vi "Visible Scrollbar.vi"(8 "error in (no error)":errorcluster, 10 "scrollbars":enum8{"hide", "show"}(ring), 11 "GObject in":refnum<vi>) -> (0 "error out":errorcluster, 1 "was scrollbars visible?":enum8{"hide", "show"}(ring), 2 "has scrollbars?":bool, 3 "GObject out":refnum<vi>)   [LabVIEW 2019, in "Builtins.lvlib"]
doc: "Shows or hides the scrollbars if it exists.\n\nCreated by: Ryan Pacini"
uses:
  Builtins.lvlib
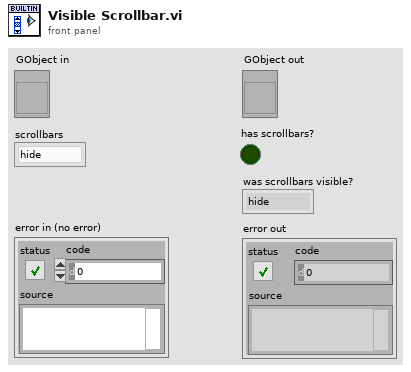
[diagram p1: front panel]
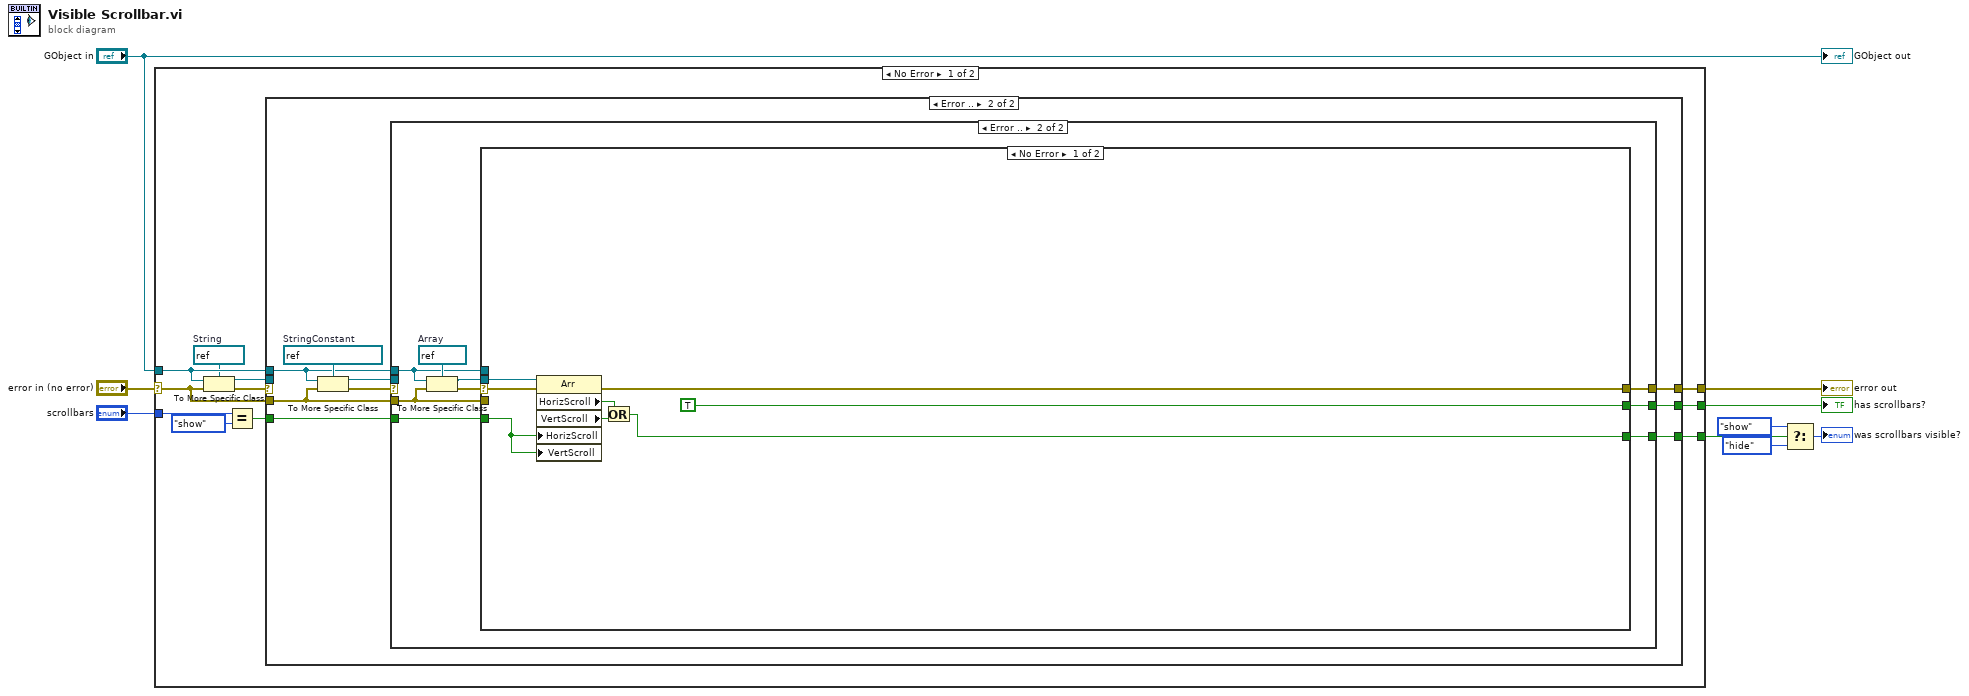
[diagram p0: block diagram]
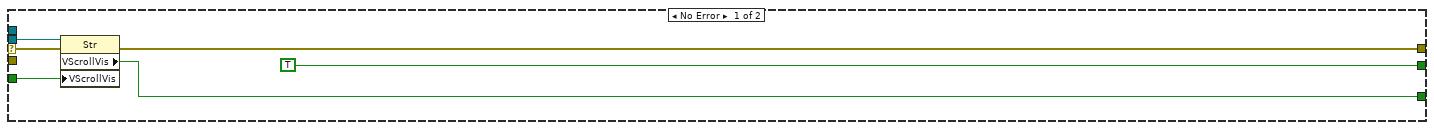
[diagram p2: hidden frame]
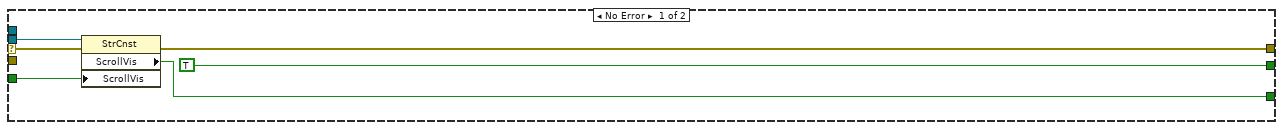
[diagram p3: hidden frame]
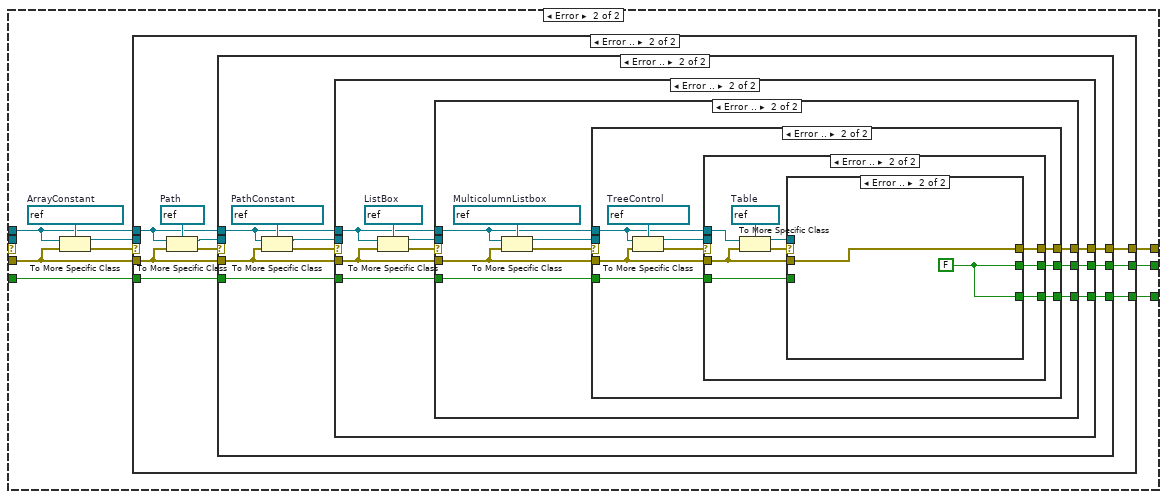
[diagram p4: hidden frame]
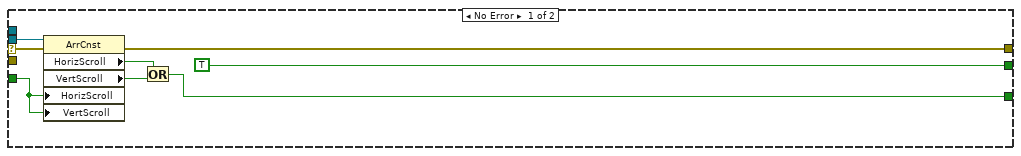
[diagram p5: hidden frame]
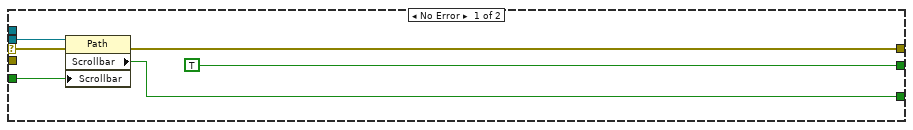
[diagram p6: hidden frame]
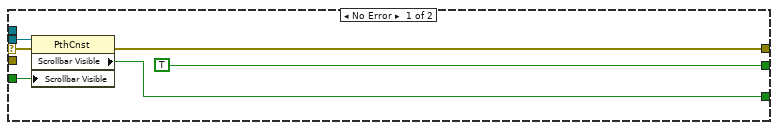
[diagram p7: hidden frame]
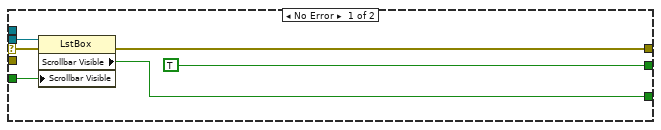
[diagram p8: hidden frame]
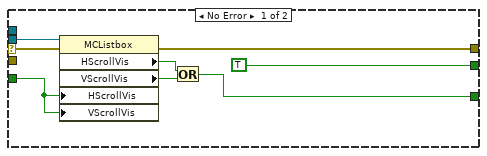
[diagram p9: hidden frame]
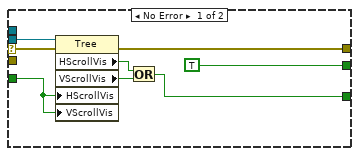
[diagram p10: hidden frame]
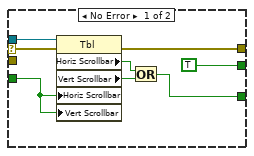
[diagram p11: hidden frame]
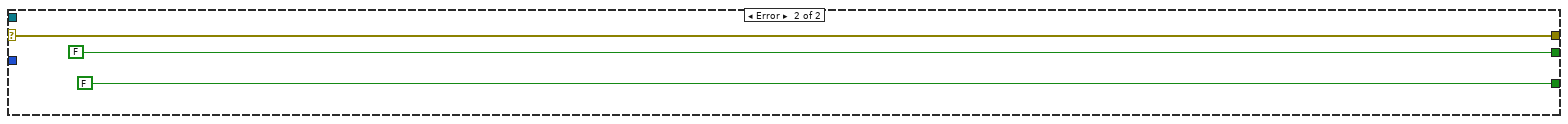
[diagram p12: hidden frame]
diagram:
  n1 = case shown="No Error" "error in (no error)" {
    selector: "error in (no error)" -> [w18 w176]
    tunnel: "GObject in" -> [w19 _]
    tunnel: "scrollbars" -> [w15 _]
    tunnel: [w20 w176] -> w7
    tunnel: [w17 FALSE] -> w6
    tunnel: [w16 FALSE ("ScrollVis")] -> w4
    frame No Error {
      w12 = refnum<vi> refnum  # String
      n2 = To More Specific Class(target class=w12, reference=w19, error in=w18) -> (specific class reference=w10:refnum<vi>, error out=w11:errorcluster)
      n3 = Equal?(x=w15, y=enum8{"hide", "show"}."show") -> (x = y?=w13:bool)
      n4 = case shown="Error .." w11 {
        selector: w11 -> [w25 _]
        tunnel: w10 -> [w24 _]
        tunnel: w13 -> [w23 w32]
        tunnel: [w22 w30] -> w20
        tunnel: w18 -> [_ w29]
        tunnel: [TRUE w31] -> w17
        tunnel: w19 -> [_ w27]
        tunnel: [w21 w28] -> w16
        frame No Error {
          n5 = property class="Str"(reference=w24, error in=w25, "VScrollVis"=w23) -> (error out=w22:errorcluster, "VScrollVis"=w21:bool)  [unwired: 1 out]
        }
        frame Error {
          w35 = refnum<vi> refnum  # StringConstant
          n6 = To More Specific Class(target class=w35, reference=w27, error in=w29) -> (specific class reference=w33:refnum<vi>, error out=w34:errorcluster)
          n7 = case shown="Error .." w34 {
            selector: w34 -> [w41 _]
            tunnel: w33 -> [w40 _]
            tunnel: w32 -> [w39 w45]
            tunnel: [TRUE w50] -> w31
            tunnel: [w37 w44] -> w30
            tunnel: w29 -> [_ w43]
            tunnel: [w36 w49] -> w28
            tunnel: w27 -> [_ w42]
            frame No Error {
              n8 = property class="StrCnst"(reference=w40, error in=w41, "ScrollVis"=w39) -> (error out=w37:errorcluster, "ScrollVis"=w36:bool)  [unwired: 1 out]
            }
            frame Error {
              w48 = refnum<vi> refnum  # Array
              n9 = To More Specific Class(target class=w48, reference=w42, error in=w43) -> (specific class reference=w46:refnum<vi>, error out=w47:errorcluster)
              n10 = case shown="No Error" w47 {
                selector: w47 -> [w57 _]
                tunnel: [TRUE w62] -> w50
                tunnel: [w53 w63] -> w49
                tunnel: w46 -> [w56 _]
                tunnel: w45 -> [w52 w64]
                tunnel: [w51 w60] -> w44
                tunnel: w43 -> [_ w61]
                tunnel: w42 -> [_ w59]
                frame No Error {
                  n11 = property class="Arr"(reference=w56, error in=w57, "HorizScroll"=w52, "VertScroll"=w52) -> (error out=w51:errorcluster, "HorizScroll"=w55:bool, "VertScroll"=w54:bool)  [unwired: 1 out]
                  n12 = Or(x=w55, y=w54) -> (x .or. y?=w53:bool)
                }
                frame Error {
                  w67 = refnum<vi> refnum  # ArrayConstant
                  n13 = To More Specific Class(target class=w67, reference=w59, error in=w61) -> (specific class reference=w65:refnum<vi>, error out=w66:errorcluster)
                  n14 = case shown="Error .." w66 {
                    selector: w66 -> [w73 _]
                    tunnel: w65 -> [w72 _]
                    tunnel: w64 -> [w71 w79]
                    tunnel: [w70 w81] -> w63
                    tunnel: [TRUE w80] -> w62
                    tunnel: w61 -> [_ w77]
                    tunnel: [w68 w78] -> w60
                    tunnel: w59 -> [_ w76]
                    frame No Error {
                      n15 = property class="ArrCnst"(reference=w72, error in=w73, "HorizScroll"=w71, "VertScroll"=w71) -> (error out=w68:errorcluster, "HorizScroll"=w75:bool, "VertScroll"=w74:bool)  [unwired: 1 out]
                      n16 = Or(x=w75, y=w74) -> (x .or. y?=w70:bool)
                    }
                    frame Error {
                      w84 = refnum<vi> refnum  # Path
                      n17 = To More Specific Class(target class=w84, reference=w76, error in=w77) -> (specific class reference=w82:refnum<vi>, error out=w83:errorcluster)
                      n18 = case shown="Error .." w83 {
                        selector: w83 -> [w90 _]
                        tunnel: w82 -> [w89 _]
                        tunnel: [w88 w96] -> w81
                        tunnel: [TRUE w94] -> w80
                        tunnel: w79 -> [w86 w95]
                        tunnel: [w85 w93] -> w78
                        tunnel: w77 -> [_ w92]
                        tunnel: w76 -> [_ w91]
                        frame No Error {
                          n19 = property class="Path"(reference=w89, error in=w90, "Scrollbar"=w86) -> (error out=w85:errorcluster, "Scrollbar"=w88:bool)  [unwired: 1 out]
                        }
                        frame Error {
                          w99 = refnum<vi> refnum  # PathConstant
                          n20 = To More Specific Class(target class=w99, reference=w91, error in=w92) -> (specific class reference=w97:refnum<vi>, error out=w98:errorcluster)
                          n21 = case shown="Error .." w98 {
                            selector: w98 -> [w105 _]
                            tunnel: w97 -> [w104 _]
                            tunnel: [w103 w110] -> w96
                            tunnel: w95 -> [w102 w111]
                            tunnel: [TRUE w109] -> w94
                            tunnel: [w100 w108] -> w93
                            tunnel: w92 -> [_ w107]
                            tunnel: w91 -> [_ w106]
                            frame No Error {
                              n22 = property class="PthCnst"(reference=w104, error in=w105, "Scrollbar Visible"=w102) -> (error out=w100:errorcluster, "Scrollbar Visible"=w103:bool)  [unwired: 1 out]
                            }
                            frame Error {
                              w114 = refnum<vi> refnum  # ListBox
                              n23 = To More Specific Class(target class=w114, reference=w106, error in=w107) -> (specific class reference=w112:refnum<vi>, error out=w113:errorcluster)
                              n24 = case shown="Error .." w113 {
                                selector: w113 -> [w120 _]
                                tunnel: w112 -> [w119 _]
                                tunnel: w111 -> [w118 w123]
                                tunnel: [w117 w126] -> w110
                                tunnel: [TRUE w125] -> w109
                                tunnel: [w115 w124] -> w108
                                tunnel: w107 -> [_ w122]
                                tunnel: w106 -> [_ w121]
                                frame No Error {
                                n25 = property class="LstBox"(reference=w119, error in=w120, "Scrollbar Visible"=w118) -> (error out=w115:errorcluster, "Scrollbar Visible"=w117:bool)  [unwired: 1 out]
                                }
                                frame Error {
                                w129 = refnum<vi> refnum  # MulticolumnListbox
                                n26 = To More Specific Class(target class=w129, reference=w121, error in=w122) -> (specific class reference=w127:refnum<vi>, error out=w128:errorcluster)
                                n27 = case shown="Error .." w128 {
                                selector: w128 -> [w137 _]
                                tunnel: w127 -> [w136 _]
                                tunnel: [w133 w143] -> w126
                                tunnel: [TRUE w142] -> w125
                                tunnel: [w131 w141] -> w124
                                tunnel: w123 -> [w130 w140]
                                tunnel: w122 -> [_ w139]
                                tunnel: w121 -> [_ w138]
                                frame No Error {
                                n28 = property class="MCListbox"(reference=w136, error in=w137, "HScrollVis"=w130, "VScrollVis"=w130) -> (error out=w131:errorcluster, "HScrollVis"=w135:bool, "VScrollVis"=w134:bool)  [unwired: 1 out]
                                n29 = Or(x=w135, y=w134) -> (x .or. y?=w133:bool)
                                }
                                frame Error {
                                w146 = refnum<vi> refnum  # TreeControl
                                n30 = To More Specific Class(target class=w146, reference=w138, error in=w139) -> (specific class reference=w144:refnum<vi>, error out=w145:errorcluster)
                                n31 = case shown="Error .." w145 {
                                selector: w145 -> [w154 _]
                                tunnel: w144 -> [w153 _]
                                tunnel: [w150 w158] -> w143
                                tunnel: [TRUE w157] -> w142
                                tunnel: [w148 w156] -> w141
                                tunnel: w140 -> [w147 w159]
                                tunnel: w139 -> [_ w155]
                                tunnel: w138 -> [_ w162]
                                frame No Error {
                                n32 = property class="Tree"(reference=w153, error in=w154, "HScrollVis"=w147, "VScrollVis"=w147) -> (error out=w148:errorcluster, "HScrollVis"=w151:bool, "VScrollVis"=w152:bool)  [unwired: 1 out]
                                n33 = Or(x=w151, y=w152) -> (x .or. y?=w150:bool)
                                }
                                frame Error {
                                w163 = refnum<vi> refnum  # Table
                                n34 = To More Specific Class(target class=w163, reference=w162, error in=w155) -> (specific class reference=w160:refnum<vi>, error out=w161:errorcluster)
                                n35 = case shown="Error .." w161 {
                                selector: w161 -> [w169 _]
                                tunnel: w160 -> [w168 _]
                                tunnel: w159 -> [w167 _]
                                tunnel: [w166 w172] -> w158
                                tunnel: [TRUE w172] -> w157
                                tunnel: [w164 w173] -> w156
                                tunnel: w155 -> [_ w173]
                                frame No Error {
                                n36 = property class="Tbl"(reference=w168, error in=w169, "Horiz Scrollbar"=w167, "Vert Scrollbar"=w167) -> (error out=w164:errorcluster, "Horiz Scrollbar"=w170:bool, "Vert Scrollbar"=w171:bool)  [unwired: 1 out]
                                n37 = Or(x=w170, y=w171) -> (x .or. y?=w166:bool)
                                }
                                frame Error {
                                w172 = FALSE
                                }
                                }
                                }
                                }
                                }
                                }
                                }
                              }
                            }
                          }
                        }
                      }
                    }
                  }
                }
              }
            }
          }
        }
      }
    }
    frame Error {
    }
  }
  "error out" <- w7
  "has scrollbars?" <- w6
  n38 = Select(t=enum8{"hide", "show"}."show" ("was inc/dec visible?"), s=w4, f=enum8{"hide", "show"}."hide" ("was inc/dec visible?")) -> (s? t:f=→"was scrollbars visible?":enum8{"hide", "show"})
  "GObject out" <- "GObject in"
